vi "Generate Velocity Vectors.vi"(9 "Nonholonomic Headings":cluster{dbl[]}[](array[cluster]), 11 "Trajectory Data In":T3(array[cluster])) -> (3 "Trajectory Data":T2(array[cluster]))   [LabVIEW 2025]
uses:
  Types/Segment Type.ctl
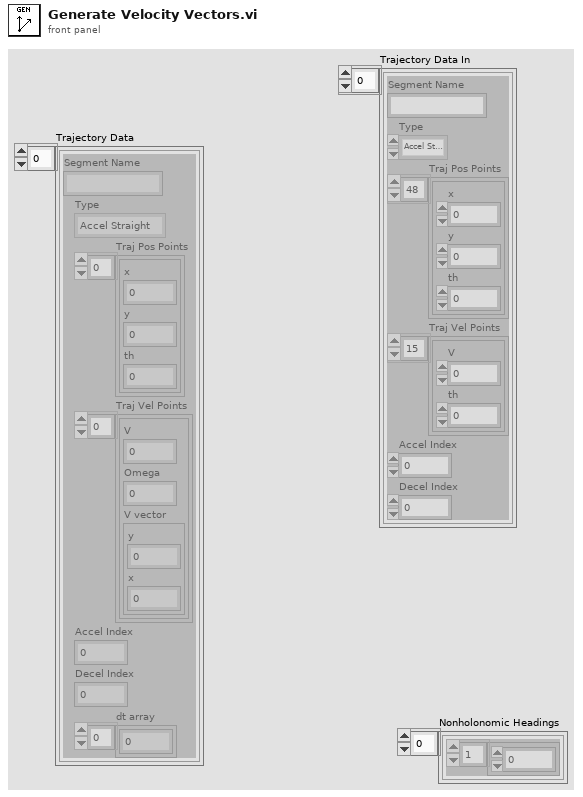
[diagram p1: front panel]
types:
  T1 = typedef "Segment Type.ctl" = enum16{"Accel Straight", "Const Straight", "Blend", "Circle", "Bezier", "Choreo"}
  T2 = cluster{"Segment Name":string, "Type":T1, "Traj Pos Points":cluster{"x":dbl, "y":dbl, "th":dbl}[], "Traj Vel Points":cluster{"V":dbl, "Omega":dbl, "V vector":cluster{"y":dbl, "x":dbl}}[], "Accel Index":i32, "Decel Index":i32, "dt array":dbl[]}[]
  T3 = cluster{"Segment Name":string, "Type":enum16{"Accel Straight", "Const Straight", "Blend", "Circle"}, "Traj Pos Points":cluster{"x":dbl, "y":dbl, "th":dbl}[], "Traj Vel Points":cluster{"V":dbl, "th":dbl}[], "Accel Index":i32, "Decel Index":i32}[]
  T4 = cluster{"Segment Name":string, "Type":T1, "Traj Pos Points":cluster{"x":dbl, "y":dbl, "th":dbl}[], "Traj Vel Points":cluster{"V":dbl, "Omega":dbl, "V vector":cluster{"y":dbl, "x":dbl}}[], "Accel Index":i32, "Decel Index":i32, "dt array":dbl[]}
  T5 = enum16{"Accel Straight", "Const Straight", "Blend", "Circle"}
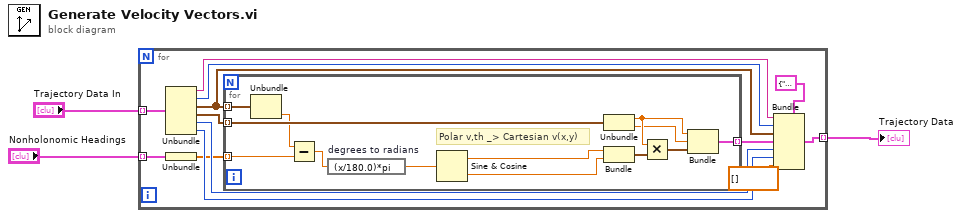
[diagram p0: block diagram]
diagram:
  n1 = for {
    tunnel: "Trajectory Data In" -> [w7] mode=indexing
    tunnel: [w16] -> w1 mode=indexing
    tunnel: "Nonholonomic Headings" -> [w6] mode=indexing
    n2 = Unbundle(w7) -> ("Segment Name"=w15:string, "Type"=w14:T5, "Traj Pos Points"=w8:cluster{"x":dbl, "y":dbl, "th":dbl}[], "Traj Vel Points"=w11:cluster{"V":dbl, "th":dbl}[], "Accel Index"=w13:i32, "Decel Index"=w12:i32)
    n3 = Unbundle(w6) -> (w9:dbl[])
    n4 = for {
      tunnel: w11 -> [w29] mode=indexing
      tunnel: w9 -> [w21] mode=indexing
      tunnel: [w25] -> w10 mode=indexing
      tunnel: w8 -> [w20] mode=indexing
      # "Polar v,th _> Cartesian v(x,y)"
      n5 = Unbundle(w20) -> ("th"=w19:dbl)  [unwired: 2 out]
      n6 = Subtract(x=w19, y=w21) -> (x-y=w22:dbl)
      n7 = expression code="(x/180.0)*pi" "degrees to radians"(w22) -> (w23:dbl)
      n8 = Sine & Cosine(0:w23) -> (1:w17:dbl, 2:w18:dbl)
      n9 = Unbundle(w29) -> ("V"=w27:dbl, "th"=w26:dbl)
      n10 = Bundle(w17, w18) -> (w28:cluster{dbl, dbl})  [unwired: 1 in]
      n11 = Multiply(x=w27, y=w28) -> (x*y=w24:cluster{dbl, dbl})
      n12 = Bundle("V"=w27, "th"=w26, w24) -> (w25:cluster{"V":dbl, "th":dbl, cluster{dbl, dbl}})  [unwired: 1 in]
    }
    n13 = Bundle(cluster=T4 {"Segment Name"="", "Type"=enum."Accel Straight", "Traj Pos Points"=[], "Traj Vel Points"=[], "Accel Index"=0, "Decel Index"=0, "dt array"=[]}, "Segment Name"=w15, "Type"=w14, "Traj Pos Points"=w8, "Traj Vel Points"=w10, "Accel Index"=w13, "Decel Index"=w12, "dt array"=dbl[] []) -> (w16:T4)
  }
  "Trajectory Data" <- w1
